vi "4_Find SN.vi"(0 "file (use dialog)":path=path "D:/20161122/LNK01E-213300ALF/Read.c") -> (3 "SN":string, 4 "Byte1":string, 6 "Byte2":string, 8 "Byte3":string, 10 "Byte4":string, 14 "SUM":string, 15 "Sum":string)   [LabVIEW 2018]
panel:
  out "array":string[][](array[string])
  out "Text file":string
  # "Byte1"
  # "Byte2"
  # "Byte3"
  # "Byte4"
  # "SUM"
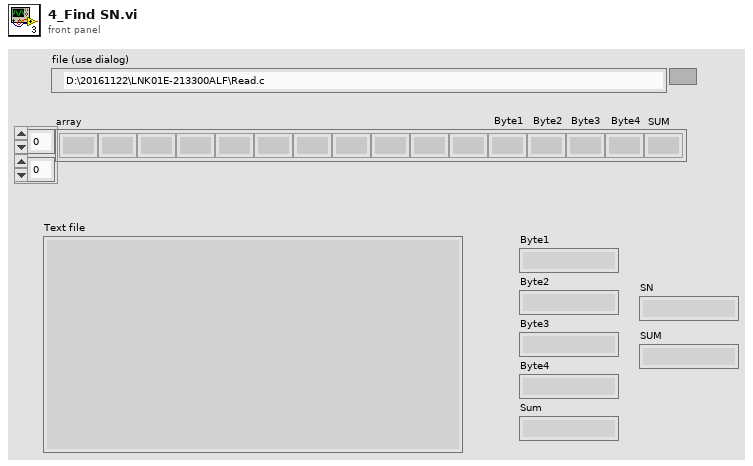
[diagram p1: front panel]
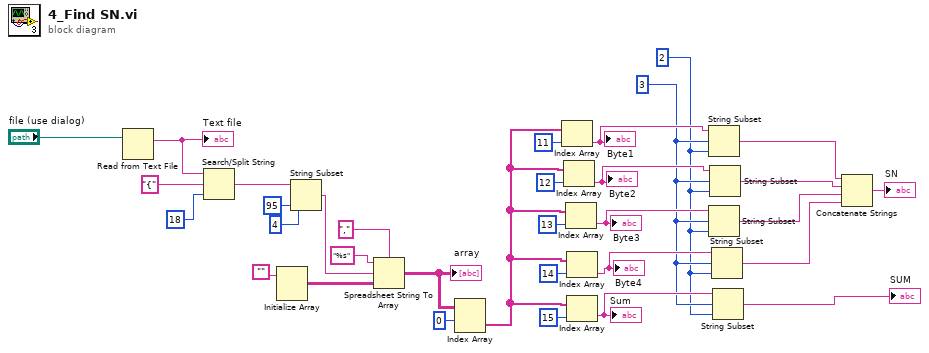
[diagram p0: block diagram]
diagram:
  w8 = 3 ("offset (0)")
  w7 = 2 ("length (rest)")
  n1 = Read from Text File(file (use dialog)="file (use dialog)") -> (text=w33:string)  [unwired: 3 in, 3 out]
  "Text file" <- w33
  n2 = Search/Split String(string=w33, search string/char (-)="{", offset (0)=18) -> (match + rest of string=w30:string)  [unwired: 2 out]
  n3 = Initialize Array("") -> (w23:string[][])  [unwired: 2 in]
  n4 = String Subset(string=w30, offset (0)=4, length (rest)=95 ("length (rest)")) -> (substring=w25:string)
  n5 = Spreadsheet String To Array(delimiter (Tab)=",", format string="%s", spreadsheet string=w25, array type (2D Dbl)=w23) -> (array=w21:string[][])
  "array" <- w21
  n6 = Index Array(array=w21, index (row)=0) -> (element=w14:string[])  [unwired: 1 in]
  n7 = Index Array(array=w14, index=11) -> (element=w13:string)
  "Byte1" <- w13
  n8 = Index Array(array=w14, index=12) -> (element=w12:string)
  "Byte2" <- w12
  n9 = Index Array(array=w14, index=13) -> (element=w11:string)
  "Byte3" <- w11
  n10 = Index Array(array=w14, index=14) -> (element=w10:string)
  "Byte4" <- w10
  n11 = Index Array(array=w14, index=15) -> (element=w9:string)
  "Sum" <- w9
  n12 = String Subset(string=w13, offset (0)=w8, length (rest)=w7) -> (substring=w6:string)
  n13 = String Subset(string=w11, offset (0)=w8, length (rest)=w7) -> (substring=w4:string)
  n14 = String Subset(string=w12, offset (0)=w8, length (rest)=w7) -> (substring=w5:string)
  n15 = String Subset(string=w10, offset (0)=w8, length (rest)=w7) -> (substring=w3:string)
  n16 = String Subset(string=w9, offset (0)=w8, length (rest)=w7) -> (substring=→"SUM":string)
  n17 = Concatenate Strings(w6, w5, w4, w3) -> (→"SN":string)
